vi "Строка TCP в кластер байт (SubVI).vi"(7 "TCP read data":string, 11 "error in":errorcluster) -> (8 "Кластер прочитанных байт":T1, 15 "error out":errorcluster)   [LabVIEW 2013]
doc: "Преобразование прочитанных даннх TCP в кластер байт"
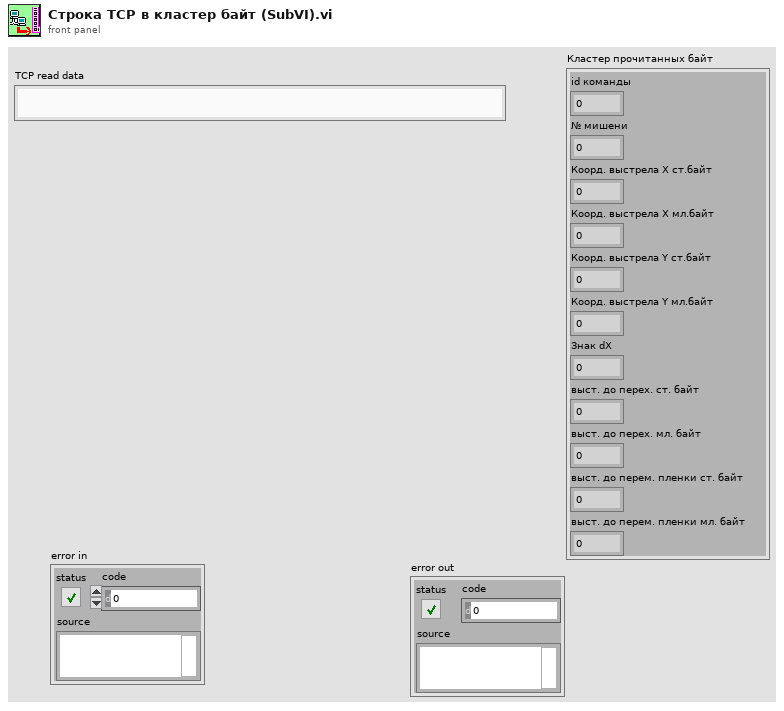
[diagram p1: front panel]
types:
  T1 = cluster{"id команды":u8, "№ мишени":u8, "Коорд. выстрела X ст.байт":u8, "Коорд. выстрела X мл.байт":u8, "Коорд. выстрела Y cт.байт":u8, "Коорд. выстрела Y мл.байт":u8, "Знак dX":i8, "выст. до перех. cт. байт":u8, "выст. до перех. мл. байт":u8, "выст. до перем. пленки ст. байт":u8, "выст. до перем. пленки мл. байт":u8}
  T2 = cluster{"id команды":u8, "№ мишени":u8, "Коорд. выстрела X ст.байт":u8, "Коорд. выстрела X мл.байт":u8, "Коорд. выстрела Y cт.байт":u8, "Коорд. выстрела Y мл.байт":u8, "Знак dX":u8, "выст. до перех. cт. байт":u8, "выст. до перех. мл. байт":u8, "выст. до перем. пленки ст. байт":u8, "выст. до перем. пленки мл. байт":u8}
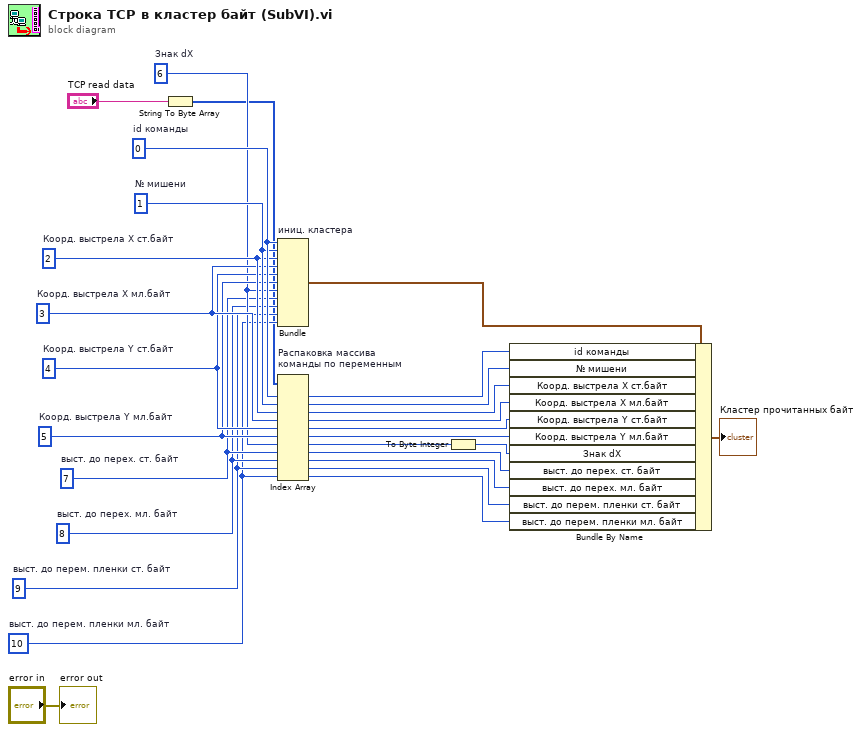
[diagram p0: block diagram]
diagram:
  w6 = u8 10  # выст. до перем. пленки мл. байт
  w7 = u8 9  # выст. до перем. пленки ст. байт
  w8 = u8 8  # выст. до перех. мл. байт
  w9 = u8 7  # выст. до перех. cт. байт
  w10 = u8 6  # Знак dX
  w11 = u8 5  # Коорд. выстрела Y мл.байт
  w12 = u8 4  # Коорд. выстрела Y cт.байт
  w13 = u8 3  # Коорд. выстрела X мл.байт
  w14 = u8 2  # Коорд. выстрела X ст.байт
  w15 = u8 1  # № мишени
  w16 = u8 0  # id команды
  n1 = String To Byte Array(string="TCP read data") -> (unsigned byte array=w1:u8[])
  n2 = Bundle "иниц. кластера"("id команды"=w16, "№ мишени"=w15, "Коорд. выстрела X ст.байт"=w14, "Коорд. выстрела X мл.байт"=w13, "Коорд. выстрела Y cт.байт"=w12, "Коорд. выстрела Y мл.байт"=w11, "Знак dX"=w10, "выст. до перех. cт. байт"=w9, "выст. до перех. мл. байт"=w8, "выст. до перем. пленки ст. байт"=w7, "выст. до перем. пленки мл. байт"=w6) -> (w4:T2)  [unwired: 1 in]
  n3 = Index Array "Распаковка массива\nкоманды по переменным"(array=w1, index #1=w16, index #2=w15, index #3=w14, index #4=w13, index #5=w12, index #6=w11, index #7=w10, index #8=w9, index #9=w8, index #10=w7, index #11=w6) -> (element #1=w27:u8, element #2=w26:u8, element #3=w25:u8, element #4=w24:u8, element #5=w23:u8, element #6=w22:u8, element #7=w21:u8, element #8=w20:u8, element #9=w19:u8, element #10=w18:u8, element #11=w17:u8)
  n4 = To Byte Integer(number=w21) -> (8bit integer=w2:i8)
  n5 = Bundle By Name(cluster=w4, "id команды"=w27, "№ мишени"=w26, "Коорд. выстрела X ст.байт"=w25, "Коорд. выстрела X мл.байт"=w24, "Коорд. выстрела Y cт.байт"=w23, "Коорд. выстрела Y мл.байт"=w22, "Знак dX"=w2, "выст. до перех. cт. байт"=w20, "выст. до перех. мл. байт"=w19, "выст. до перем. пленки ст. байт"=w18, "выст. до перем. пленки мл. байт"=w17) -> (→"Кластер прочитанных байт":T2)
  "error out" <- "error in"
